vi "VdDigitalControl_AdvantechADAM_Create.vi"(8 "Error In":errorcluster, 10 "Address":string, 11 "reference in":refnum<class "VdDigitalControl_AdvantechADAM.lvclass">) -> (0 "Error Out":errorcluster, 3 "reference out":refnum<class "VdDigitalControl_AdvantechADAM.lvclass">)   [LabVIEW 2020, in "VdDigitalControl_AdvantechADAM.lvclass"]
uses:
  VdDigitalControl_AdvantechADAM.lvclass
  VdDigitalControl_AdvantechADAM.lvclass/VdDigitalControl_AdvantechADAM.ctl
  VdDigitalControl_class/VdDigitalControl.lvclass
  <vilib>/Instr/_visa.llb/VISA Configure Serial Port (Instr).vi
  C:/Projects/OpenGDS_DesignPatterns/Factory1/VdDigitalControl_class/VdDigitalControl.lvclass
  C:/Projects/OpenGDS_DesignPatterns/Factory1/VdInstrument_class/VdInstrument.lvclass
  C:/Projects/OpenGDS_DesignPatterns/Factory1/VdDigitalControl_AdvantechADAM_class/VdDigitalControl_AdvantechADAM.lvclass
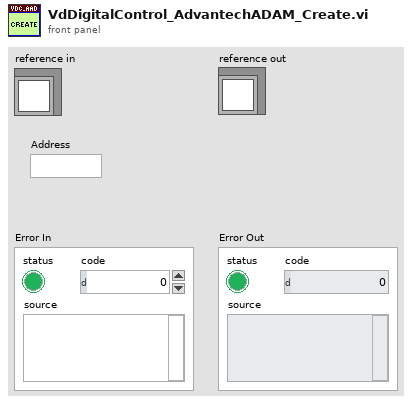
[diagram p1: front panel]
types:
  T1 = typedef "VdDigitalControl_AdvantechADAM.lvclass/ObjectAttributes.ctl" = cluster{"VISARef":refnum<visa-resource-name>}
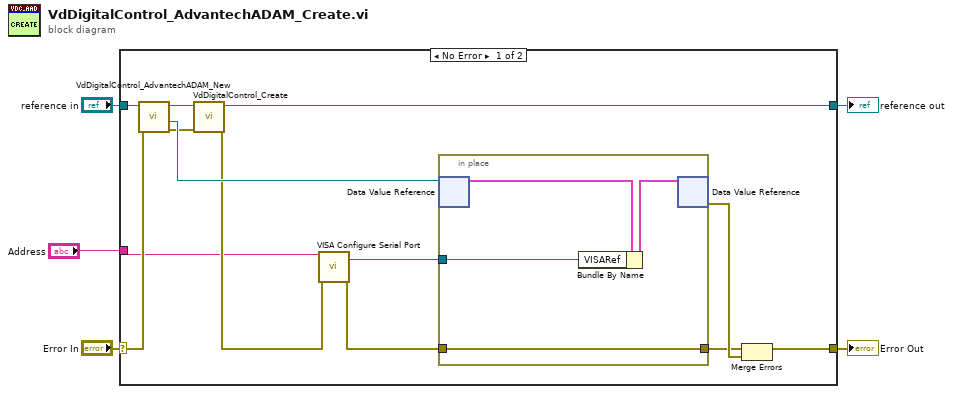
[diagram p0: block diagram]
diagram:
  n1 = case shown="No Error" "Error In" {
    selector: "Error In" -> [w14 w24]
    tunnel: [w12 w24] -> w4
    tunnel: "reference in" -> [w16 w23]
    tunnel: [w11 w23] -> w2
    tunnel: "Address" -> [w6 _]
    frame No Error {
      n2 = call "VdDigitalControl_AdvantechADAM_New.vi"("error in (no error)"=w14, "reference in"=w16) -> ("error out"=w15:errorcluster, "DVRRefOut"=w18:refnum<data-value>, "reference out"=w17:refnum<class "VdDigitalControl_AdvantechADAM.lvclass">)  [unwired: 6 in, 1 out]
      n3 = call "VdDigitalControl_Create.vi"("Error In"=w15, "reference in"=w17) -> ("Error Out"=w9:errorcluster, "reference out"=w11:refnum<class "VdDigitalControl_AdvantechADAM.lvclass">)  [unwired: 8 in]
      n4 = call-poly "VISA Configure Serial Port"("VISA resource name"=w6, "error in (no error)"=w9) -> ("VISA resource name out"=w7:refnum<visa-resource-name>, "error out"=w8:errorcluster)  [unwired: 12 in]
      n5 = in-place {
        in-place-border: w8 -> [w20]
        in-place-border: [w20] -> w10
        in-place-border: w7 -> [w19]
        n6 = in-place-dvr #1(w18) -> (w21:T1)  [unwired: 1 out]
        n7 = Bundle By Name(cluster=w21, "VISARef"=w19) -> (w22:T1)
        n8 = in-place-dvr #1(w22) -> (w13:errorcluster)  [unwired: 1 out]
      }
      n9 = Merge Errors(w10, w13) -> (w12:errorcluster)
    }
    frame Error {
    }
  }
  "Error Out" <- w4
  "reference out" <- w2
